vi "clickInsideImage.vi"(8 "error in (no error)":errorcluster, 10 "Point":T1, 11 "ImageStreamViewer in":refnum<class "ImageStreamViewer.lvclass">) -> (0 "error out":errorcluster, 2 "clickInsideImage?":bool, 3 "ImageStreamViewer out":refnum<class "ImageStreamViewer.lvclass">)   [LabVIEW 2011, in "Views.lvlib" / "Camera.lvlib" / "ImageStreamViewer.lvclass"]
uses:
  ImageStreamViewer.lvclass
  <vilib>/Utility/miscctls.llb/LVPoint32TypeDef.ctl
  ImageStreamViewer.lvclass/ImageStreamViewer.ctl
panel:
  # "Was the click inside the image, or only on the image frame?"
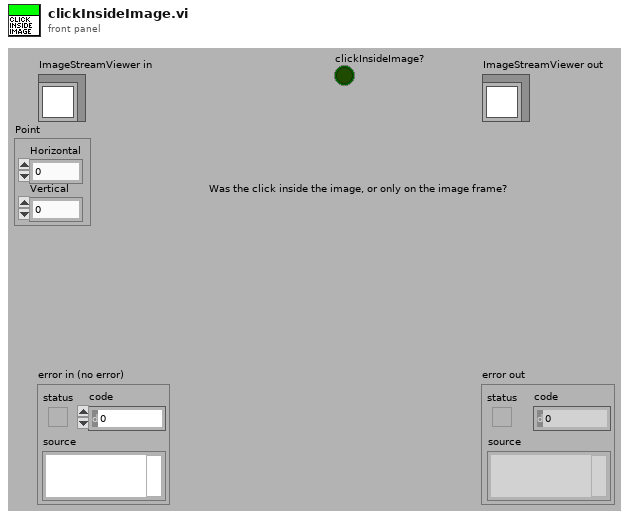
[diagram p1: front panel]
types:
  T1 = typedef "LVPoint32TypeDef.ctl" = cluster{"Horizontal":i32, "Vertical":i32}
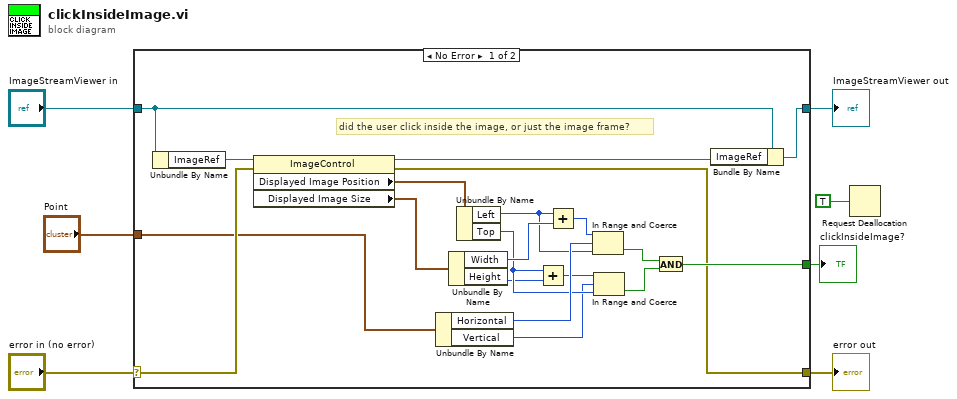
[diagram p0: block diagram]
diagram:
  n1 = case shown="No Error" "error in (no error)" {
    selector: "error in (no error)" -> [w26 w29]
    tunnel: [w9 w29] -> w6
    tunnel: [w10 w28] -> w4
    tunnel: "ImageStreamViewer in" -> [w11 w28]
    tunnel: [w13 _] -> w3
    tunnel: "Point" -> [w8 _]
    frame No Error {
      # "did the user click inside the image, or just the image frame?"
      n2 = Unbundle By Name(w11) -> ("ImageRef"=w27:refnum<vi>)
      n3 = property class="ImageControl"(reference=w27, error in=w26) -> (reference out=w12:refnum<vi>, error out=w9:errorcluster, "Displayed Image Position"=w25:cluster{"Left":i32, "Top":i32}, "Displayed Image Size"=w24:cluster{"Width":u32, "Height":u32})
      n4 = Unbundle By Name(w8) -> ("Horizontal"=w23:i32, "Vertical"=w16:i32)
      n5 = Unbundle By Name(w24) -> ("Width"=w21:u32, "Height"=w17:u32)
      n6 = Unbundle By Name(w25) -> ("Left"=w20:i32, "Top"=w18:i32)
      n7 = Add(x=w18, y=w17) -> (x+y=w19:u32)
      n8 = Add(x=w20, y=w21) -> (x+y=w22:u32)
      n9 = In Range and Coerce(upper limit=w22, x=w23, lower limit=w20) -> (In Range?=w15:bool)  [unwired: 1 out]
      n10 = In Range and Coerce(upper limit=w19, x=w16, lower limit=w18) -> (In Range?=w14:bool)  [unwired: 1 out]
      n11 = And(x=w15, y=w14) -> (x .and. y?=w13:bool)
      n12 = Bundle By Name(cluster=w11, "ImageRef"=w12) -> (w10:refnum<class "ImageStreamViewer.lvclass">)
    }
    frame Error {
    }
  }
  "error out" <- w6
  "ImageStreamViewer out" <- w4
  "clickInsideImage?" <- w3
  n13 = Request Deallocation(TRUE ("flag")) -> ()
